vi "call-C-proj.vi"(6 "error in":errorcluster, 7 "ball size":i32=13, 8 "Ymax":i32=405, 9 "Ymin":i32=102, 10 "Xmax":i32=740, 11 "Xmin":i32=127) -> (0 "white":cluster{i32, i32, i32}={137, 177, 138}, 1 "yellow":cluster{i32, i32, i32}={369, 284, 85}, 2 "red":cluster{i32, i32, i32}={-1, -1, 0}, 3 "erreur call C":errorcluster, 4 "Warnings C":string="Warning : seulement 2 boule(s) trouvee(s) sur 3.\n", 5 "erreur C":errorcluster)   [LabVIEW 2025]
panel:
  out "C data":string
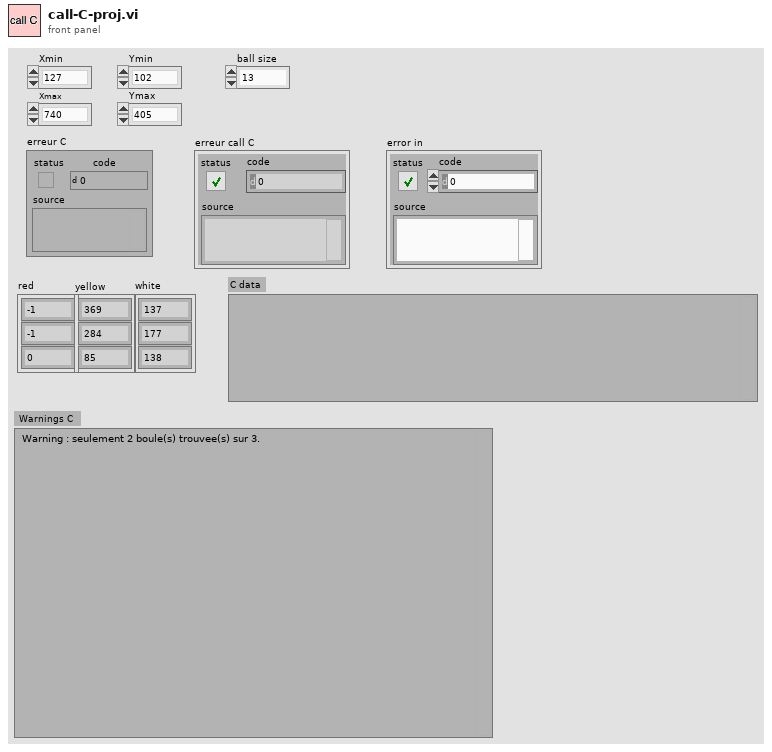
[diagram p1: front panel]
types:
  T1 = enum16{"open", "replace", "create", "open or create", "replace or create", "replace or create with confirmation"}
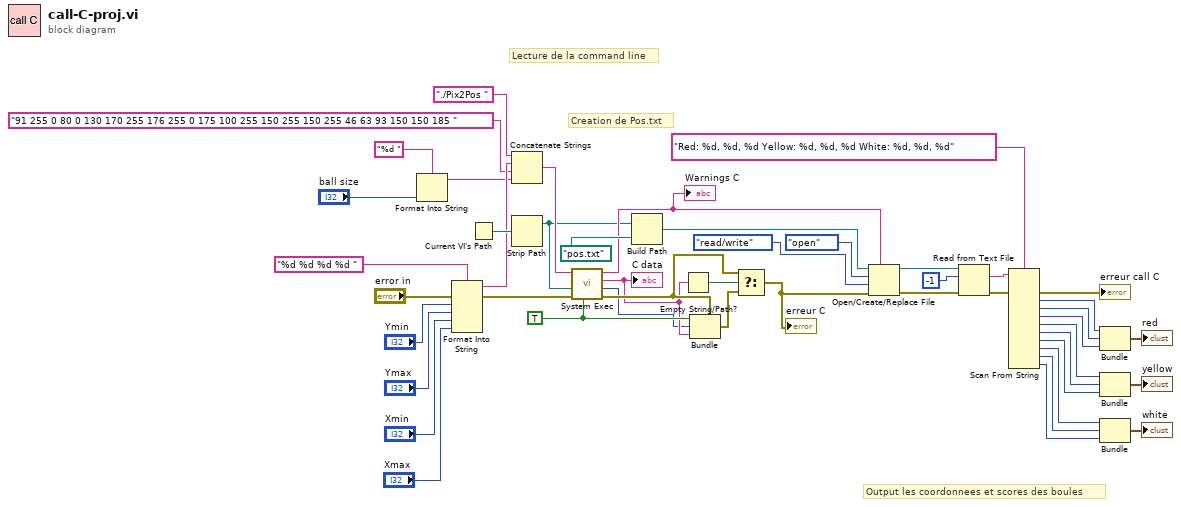
[diagram p0: block diagram]
diagram:
  w4 = TRUE
  # "Output les coordonnees et scores des boules"
  # "Creation de Pos.txt"
  # "Lecture de la command line"
  n1 = Format Into String(format string="%d ", "ball size") -> (resulting string=w11:string)  [unwired: 2 in, 1 out]
  n2 = Format Into String(format string="%d %d %d %d ", error in="error in", "Ymin", "Ymax", "Xmin", "Xmax") -> (resulting string=w15:string, error out=w10:errorcluster)  [unwired: 1 in]
  n3 = Current VI's Path() -> (path=w46:path)
  n4 = Concatenate Strings("./Pix2Pos " ("string"), w15, "91 255 0 80 0 130 170 255 176 255 0 175 100 255 150 255 150 255 46 63 93 150 150 185 " ("string"), w11) -> (w47:string)
  n5 = Strip Path(path=w46) -> (stripped path=w21:path)  [unwired: 1 out]
  n6 = call <vilib>:"System Exec.vi"("run minimized? (F)"=w4, "error in (no error)"=w10, "working directory"=w21, "command line"=w47) -> ("error out"=w5:errorcluster, "return code"=w2:i32, "standard error"=w3:string, "standard output"=w23:string)  [unwired: 4 in]
  "C data" <- w3
  "Warnings C" <- w23
  n7 = Build Path(base path=w21, name or relative path=path "pos.txt") -> (appended path=w24:path)
  n8 = Empty String/Path?(string/path=w3) -> (empty?=w7:bool)
  n9 = Bundle(cluster=w5, "status"=w4, "code"=w2, "source"=w3) -> (w6:errorcluster)
  n10 = Select(t=w5, s=w7, f=w6) -> (s? t:f=w1:errorcluster)
  "erreur C" <- w1
  n11 = Open/Create/Replace File(file path (use dialog)=w24, error in=w1, prompt=w23, operation (0:open)=T1."open", access (0:read/write)=enum16{"read/write", "read-only", "write-only"}."read/write") -> (refnum out=w41:refnum<file>, error out=w40:errorcluster)  [unwired: 1 in, 1 out]
  n12 = Read from Text File(file (use dialog)=w41, count=-1, error in=w40) -> (text=w42:string, error out=w39:errorcluster)  [unwired: 1 in, 2 out]
  n13 = Scan From String(format string="Red: %d, %d, %d Yellow: %d, %d, %d White: %d, %d, %d", input string=w42, error in=w39) -> (error out=→"erreur call C":errorcluster, output 1=w38:i32, output 2=w37:i32, output 3=w36:i32, output 4=w35:i32, output 5=w34:i32, output 6=w33:i32, output 7=w32:i32, output 8=w31:i32, output 9=w30:i32)  [unwired: 10 in, 2 out]
  n14 = Bundle(w38, w37, w36) -> (→"red":cluster{i32, i32, i32})  [unwired: 1 in]
  n15 = Bundle(w35, w34, w33) -> (→"yellow":cluster{i32, i32, i32})  [unwired: 1 in]
  n16 = Bundle(w32, w31, w30) -> (→"white":cluster{i32, i32, i32})  [unwired: 1 in]
